vi "Set_Tree_Item_Source_Contained_File.vi"(8 "error in (no error)":errorcluster, 10 "data":T1, 11 "IB_TreeCtrFileItem in":refnum<class "IB_Tree_Item_Source_Contained_File.lvclass">) -> (0 "error out":errorcluster, 3 "IB_TreeCtrFileItem out":refnum<class "IB_Tree_Item_Source_Contained_File.lvclass">)   [LabVIEW 2020, in "IB_Tree_Item_Source_Contained_File.lvclass"]
uses:
  <vilib>/AppBuilder/IB_Classes/Tree_Item_Source_Contained_File/IB_Tree_Item_Source_Contained_File.lvclass
  <vilib>/AppBuilder/IB_Classes/Tree_Item_Source_Contained_File/IB_Tree_Item_Source_Contained_File.lvclass/IB_Tree_Item_Source_Contained_File.ctl
  <vilib>/AppBuilder/IB_Classes/Tree_Item_Virtual_Folder/IB_Tree_Item_Virtual_Folder.lvclass
  <vilib>/AppBuilder/IB_Classes/Tree_Item_Source_Contained_File/IB_Tree_Item_Source_Contained_File.ctl
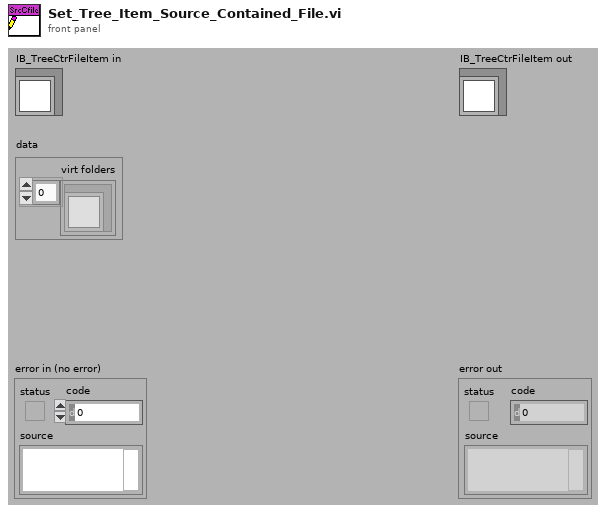
[diagram p1: front panel]
types:
  T1 = typedef "IB_Tree_Item_Source_Contained_File.ctl" = cluster{"virt folders":refnum<class "IB_Tree_Item_Virtual_Folder.lvclass">[]}
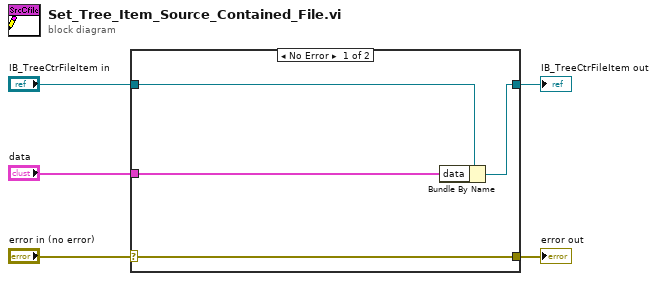
[diagram p0: block diagram]
diagram:
  n1 = case shown="No Error" "error in (no error)" {
    selector: "error in (no error)" -> [w9 w10]
    tunnel: [w9 w10] -> w4
    tunnel: [w7 w11] -> w2
    tunnel: "IB_TreeCtrFileItem in" -> [w8 w11]
    tunnel: "data" -> [w6 _]
    frame No Error {
      n2 = Bundle By Name(cluster=w8, "data"=w6) -> (w7:refnum<class "IB_Tree_Item_Source_Contained_File.lvclass">)
    }
    frame Error {
    }
  }
  "error out" <- w4
  "IB_TreeCtrFileItem out" <- w2
